vi "Remove Tagged Sections.vi"() -> ()   [LabVIEW 2024]
panel:
  out "string out":string
  in  "open tag":string
  in  "close tag":string
  in  "string":string
  # "~-mul(858,892)?@#mul(380,985)what()[^what()%mul(340,11)~*}don't())/~-mul(849,387)%-why()when():how()>-,what()mul(605,504)what()~:]what();how()who()];mul(771,783)?^ who()}~?>mul(111,830))@ ~mul(329,797)%'why()why()mul(125,409)-*/where()()@&!why()mul(390,37)when(974,538)#/when()){/don't()/mul(20,990)}?%{(who()mul(627,567)(how()'<(#%how()mul(387,315){;%who()%#from()mul(868,680)}^$mul(862,19)mul(847,689)>((#@when()}mul(339,156)+/{}@{^%[why(231,704)mul(236,754)]'^where(978,690)mul(460,872)#'*mul(518,944)>mul(301,886))mul(477,933)^mul(685,909)who())]what(288,791)mul(170,434){ &where()~(@where()mul(191,104)mul(637,600)&select()why())~select()mul(534,617)?mul(763,508){from()when(22,266)+who() when()mul(204,352)when()mul(426,122)-<*where()'$ why()mul(192,980)[(#[!$-}mul(798,208)''[!where()what()select()mul(295,727))#)}($<?<mul(452,502)(don't()mul(737,492)>,$%where(539,126)what()when()select()'@mul(311,541),?don't()#select()!}!(}&?mul(100,142)),-}%mul(222,856)~$;>!from()where()mul(758,901)mul(757,796)mul(976,686);@'~+-{#who()mul(26,971);mul(404,362)^~who(417,106)what()#mul(186,691)from() %#+{/mul(67,433)-who()!-+!mul(184,469)*when()[&when(458,221)<$mul(163,556)^)]?,'}&+who()mul(514,239)~)(mul(143,441)'how(741,776)~who(766,575)when();>*^mul(281,143)+!>;+:mul(767,44)#<mul(490,849)> when()why()don't()how()from()[from()from(){mul(436,519)what() *who();@{,>do()%'mul(19,540)when()mul(643,539)~when(812,543)mul(527,639)-!mul(409,379)where()/(mul(168,491)#$>]mul(432,333)@%<when();{?what()^mul(819,413)'where(65,845)}-' ^@don't()?how()when()>><mul(591,832)where(600,755)]who()}do()!^-$what()from()select()'#mul(572,956)@#:what()from(),]mul(303,346) when()$$how()@%/#$mul(857,344)/what()where()mul(969,234)$!#when()>>&who()(mul(113,494)%where()why()when()mul(659,592)<why()!<}mul(429,162)[who()*>#(/'mul(72,670)when()^^mul(369,596)mul(631,168)-why()()[*}mul(330,968) $why()where()mul(230,139)don't()@)@<mul(849,413)-when(){*?]mul(821,9)mul(753,277)]{&when()%:mul(262,360)what()mul(65,276)don't()])who();where()$!,(-mul(952,221)+:/{where()where()mul(608,843)'>where())%}where()&,}mul(875,661)~don't()':why(){mul(793*:mul(399,702)!://select()@when()why()do()@mul(488,581{?{&<who(617,140)@how()mul(156,982)why()'&<where()*:{mul(452{-+$$*/mul(202,724)]#:#why()+??(#mul(607,2)@^mul(20,845)#{+#[/#~/mul(111,872)how()select()]<how())'how()mul(921,254)$:;/where() ~why()}?mul(558,122)@how()<<who()mul(992,319)what(734,450)[^mul(498,490)/mul(632,639)when()]from(){why()]$[who(664,268)mul(401,695]!>how()&select()!<'mul(912,311)why()! })@+}mul(128*mul(626,752)%mul(49,60)[,who()what()select()<what()mul(24,8)>)@@]*]why(937,788)from():mul(945,658)<]don't()where()how(515,644)@+'select()how()mul(369,665)/],<when(){( $how()mul(361,594)$select()&:{:$when()mul(52,806) #from()@when()where():>mul(263,185)where()^why()why()@what()mul(82,407)mul(464,537)[mul(871,333)^mul(560,227)-why()mul(966,203)$what()+where()#mul(101,21)}%how(),)^who()>,select()mul(667,565)('what(),%select()(@mul(500,204:''<~'why(477,559)<do()>)[where()mul(698,648);how(){&?what()^@[%mul(280,395)>~, mul-#/%:where()>where():mul(170,746)don't()}($:@mul(998,876)*~<[mul(121,366)-?#;how()>from() ::mul(804,883)^-[  (:mul(100,354who(544,766)+,]>!['/;mul(949,115)"
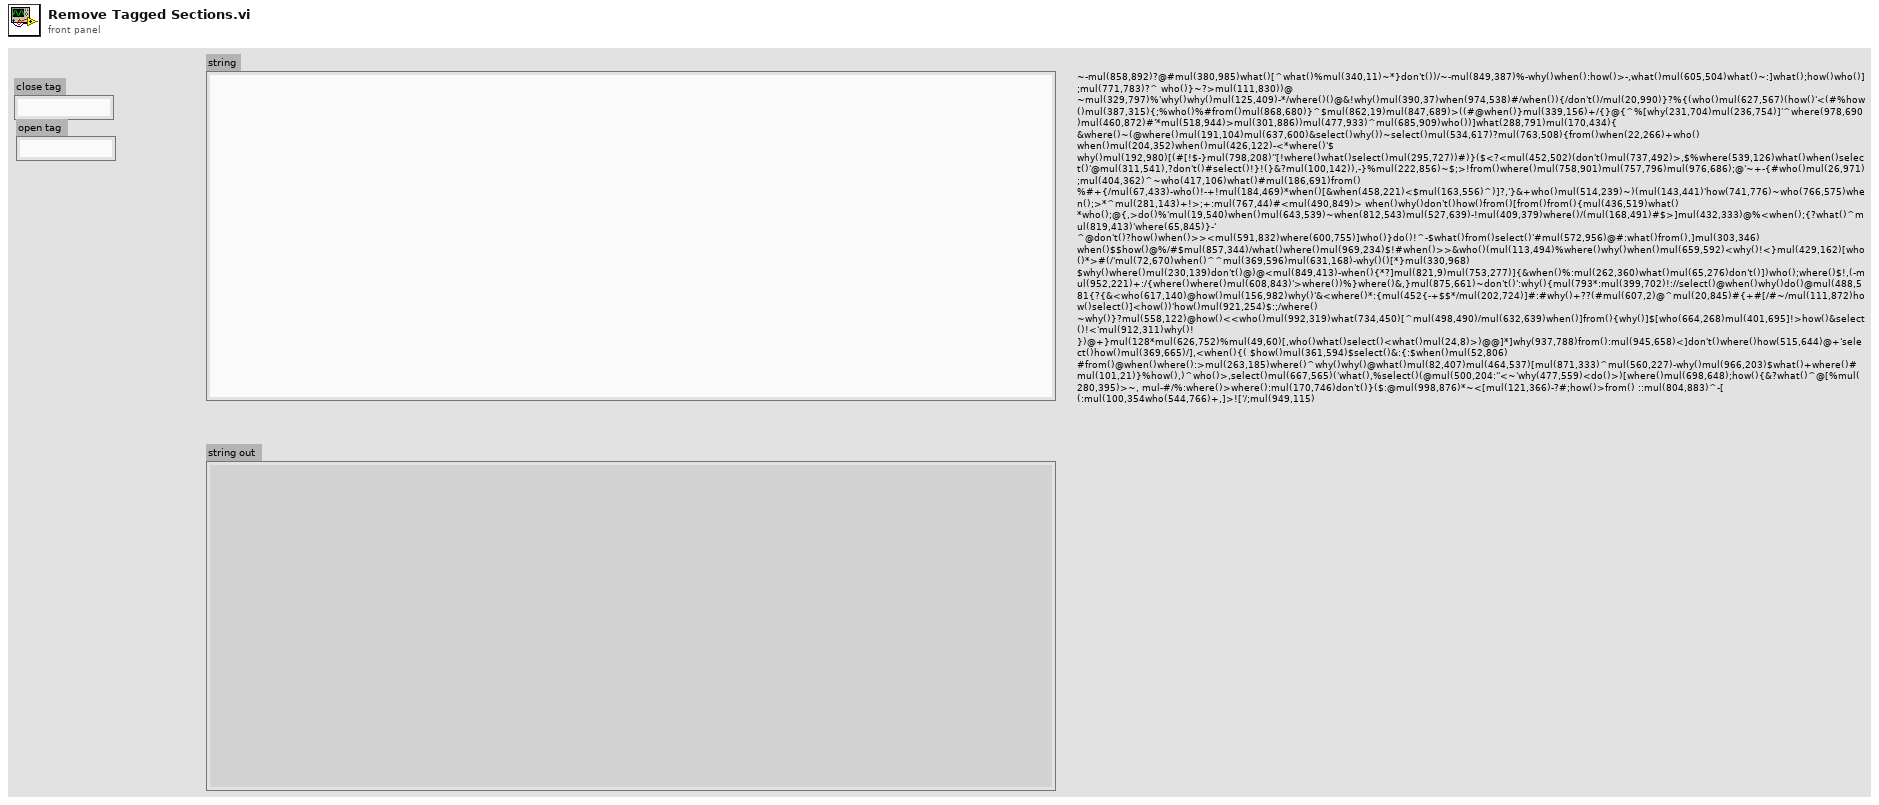
[diagram p1: front panel]
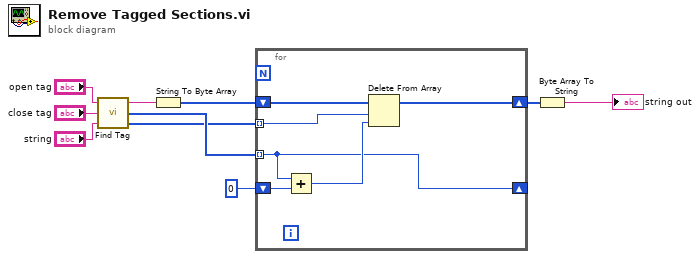
[diagram p0: block diagram]
diagram:
  n1 = call <vilib>:"Find Tag.vi"("string"="string", "close tag"="close tag", "open tag"="open tag") -> ("Length"=w5:i32[], "Start"=w6:i32[], "string out"=w7:string)
  n2 = String To Byte Array(string=w7) -> (unsigned byte array=w4:u8[])
  n3 = for {
    tunnel: w6 -> [w11] mode=indexing
    tunnel: w5 -> [w14] mode=indexing
    shift-right: [w15] -> w2
    shift-left: w4 -> [w16]
    shift-right: [w11] -> _
    shift-left: 0 -> [w12]
    n4 = Add(x=w11, y=w12) -> (x+y=w13:i32)
    n5 = Delete From Array(array=w16, length=w14, index=w13) -> (array with subset deleted=w15:u8[])  [unwired: 1 out]
  }
  n6 = Byte Array To String(unsigned byte array=w2) -> (string=→"string out":string)
